vi "氨氮测量流程.vi"(10 "量程模式":T1, 11 "参数":T2={"站号"=1, "量程切换"=enum."AUTO", "控制命令"=enum."启动测量", "模式设置"=enum."待机", "测量间隔"=0} {"站号" items=["总磷"=1, "总氮"=2]}) -> ()   [LabVIEW 2016, in "斯坦道氨氮.lvlib"]
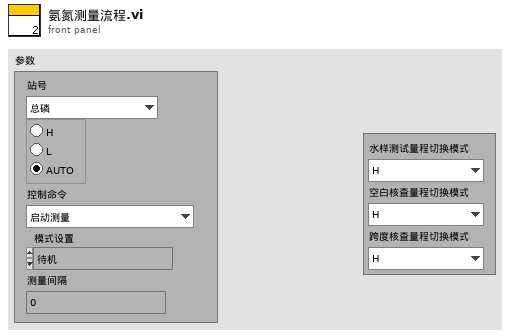
[diagram p1: front panel]
types:
  T1 = cluster{"水样测试量程切换模式":enum16{"H", "L", "AUTO"}, "空白核查量程切换模式":enum16{"H", "L", "AUTO"}, "跨度核查量程切换模式":enum16{"H", "L", "AUTO"}}
  T2 = cluster{"站号":u16, "量程切换":enum32{"H", "L", "AUTO"}, "控制命令":enum16{"启动测量", "标样核查", "零点核查", "跨度核查", "空白测试", "平行样测试", "加标回收", "空白校准", "标样校准", "初始化（清洗）", "停止测试", "仪器重启", "校时", "模式设置", "测量间隔设置"}, "模式设置":enum16{"待机", "连续模式", "周期模式", "定点模式", "受控模式", "手动模式"}, "测量间隔":u16}
  T3 = enum16{"初始化", "通电", "参数1启动", "等待参数1测试完成", "参数1测试完成", "参数1存储数据", "参数2启动", "等待参数2测试完成", "参数2测试完成", "参数2存储数据", "断电", "结束"}
  T4 = cluster{"运行模式":enum16{"维护模式", "常规模式", "应急模式", "质控模式"}, "质控频次":enum16{"关闭", "每天", "星期一", "星期二", "星期三", "星期四", "星期五", "星期六", "星期日"}, "空白核查时间":u16, "跨度核查时间":u16, "24H周期设置":bool[]}
  T5 = cluster{"时间标识":timestamp, "设备":string, "日志信息":string, "流程参数":string}
  T6 = cluster{"时间标识":timestamp, "监测值":sgl, "单位":u16, "数据标识":string, "因子编码":u32, "标样参考值":sgl, "F0":sgl, "F1":sgl, "F2":sgl, "F3":sgl, "温度":sgl, "湿度":sgl, "量程标识":string}
  T7 = enum16{"维护数据", "水样测试", "标样核查", "零点核查", "跨度核查", "空白测试", "平行样测试", "加标回收", "空白校准", "标样校准", "初始化（清洗）"}
  T8 = cluster{"系统时间":timestamp, "工作状态":enum16{"空闲", "水样测试", "标样核查", "零点核查", "跨度核查", "空白测试", "平行样测试", "加标回收", "空白校准", "标样校准", "初始化（清洗）"}, "测量模式":enum16{"待机", "连续模式", "周期模式", "定点模式", "受控模式", "手动模式"}, "告警代码":enum16{"无告警", "缺试剂告警", "缺水样告警", "缺蒸馏水告警", "缺标液告警", "仪表漏液告警", "标定异常告警", "超量程告警", "加热异常", "低试剂预警", "超上限告警", "超下限告警", "仪表内部其他异常", "滴定异常告警", "电极异常告警", "量程切换告警", "参数设置告警", "PH电极电位异常", "电导率电极异常", "浊度光度异常", "溶解氧电极异常", "溶解氧光强异常", "温度异常告警", "PH异常告警", "溶解氧异常告警", "电导率异常告警", "浊度异常告警", "叶绿素异常告警", "藻密度异常告警", "蓝绿藻异常告警", "ORP异常告警", "氨氮异常告警", "清洁刷异常告警", "SD卡异常告警", "蓝牙异常告警", "Wifi异常告警", "流程异常告警"}, "故障代码":enum16{"无故障", "电机故障", "温度故障", "通讯故障", "滴定故障"}, "日志代码":u16, "软件版本":u16, "F0":sgl, "F1":sgl, "F2":sgl, "F3":sgl, "T":sgl, "H":sgl, "id":u16, "flowid":u16, "量程":u16, "总磷控温温度1":sgl, "营养盐控温温度2":sgl, "ADC":sgl}
  T9 = enum16{"启动测量", "标样核查", "零点核查", "跨度核查", "空白测试", "平行样测试", "加标回收", "空白校准", "标样校准", "初始化（清洗）", "停止测试", "仪器重启", "校时", "模式设置", "测量间隔设置"}
  T10 = enum16{"空闲", "水样测试", "标样核查", "零点核查", "跨度核查", "空白测试", "平行样测试", "加标回收", "空白校准", "标样校准", "初始化（清洗）"}
  T11 = cluster{"跨度值":dbl, "零点标准液浓度":dbl, "跨度标准液浓度":dbl, "标准液标准浓度":dbl}
  T12 = cluster{"因子编码":u32, "单位":u16, "标样参考值":sgl, "水样数据时间":timestamp, "水样实测值":sgl, "水样数据标识":string, "标样数据时间":timestamp, "标样实测值":sgl, "标样数据标识":string, "空白数据时间":timestamp, "空白实测值":sgl, "空白数据标识":string, "零点核查数据时间":timestamp, "零点核查实测值":sgl, "零点核查数据标识":string, "跨度核查数据时间":timestamp, "跨度核查实测值":sgl, "跨度核查数据标识":string, "加标回收数据时间":timestamp, "加标回收实测值":sgl, "加标回收数据标识":string, "平行样数据时间":timestamp, "平行样实测值":sgl, "平行样数据标识":string}
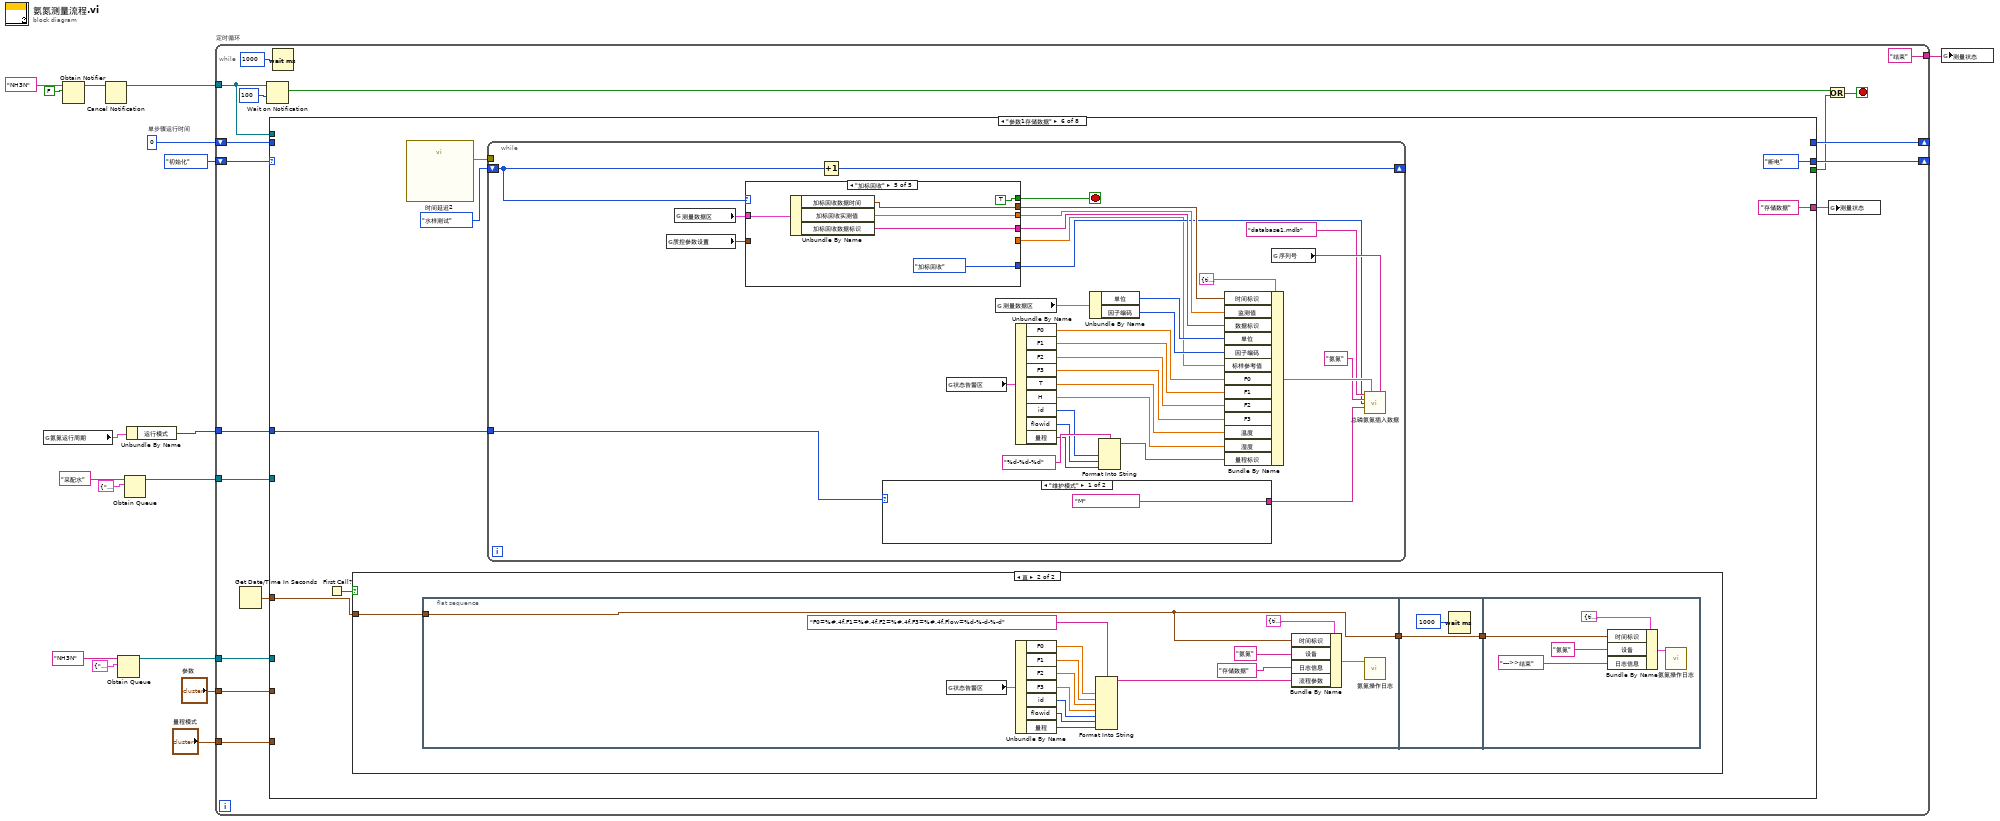
[diagram p0: block diagram]
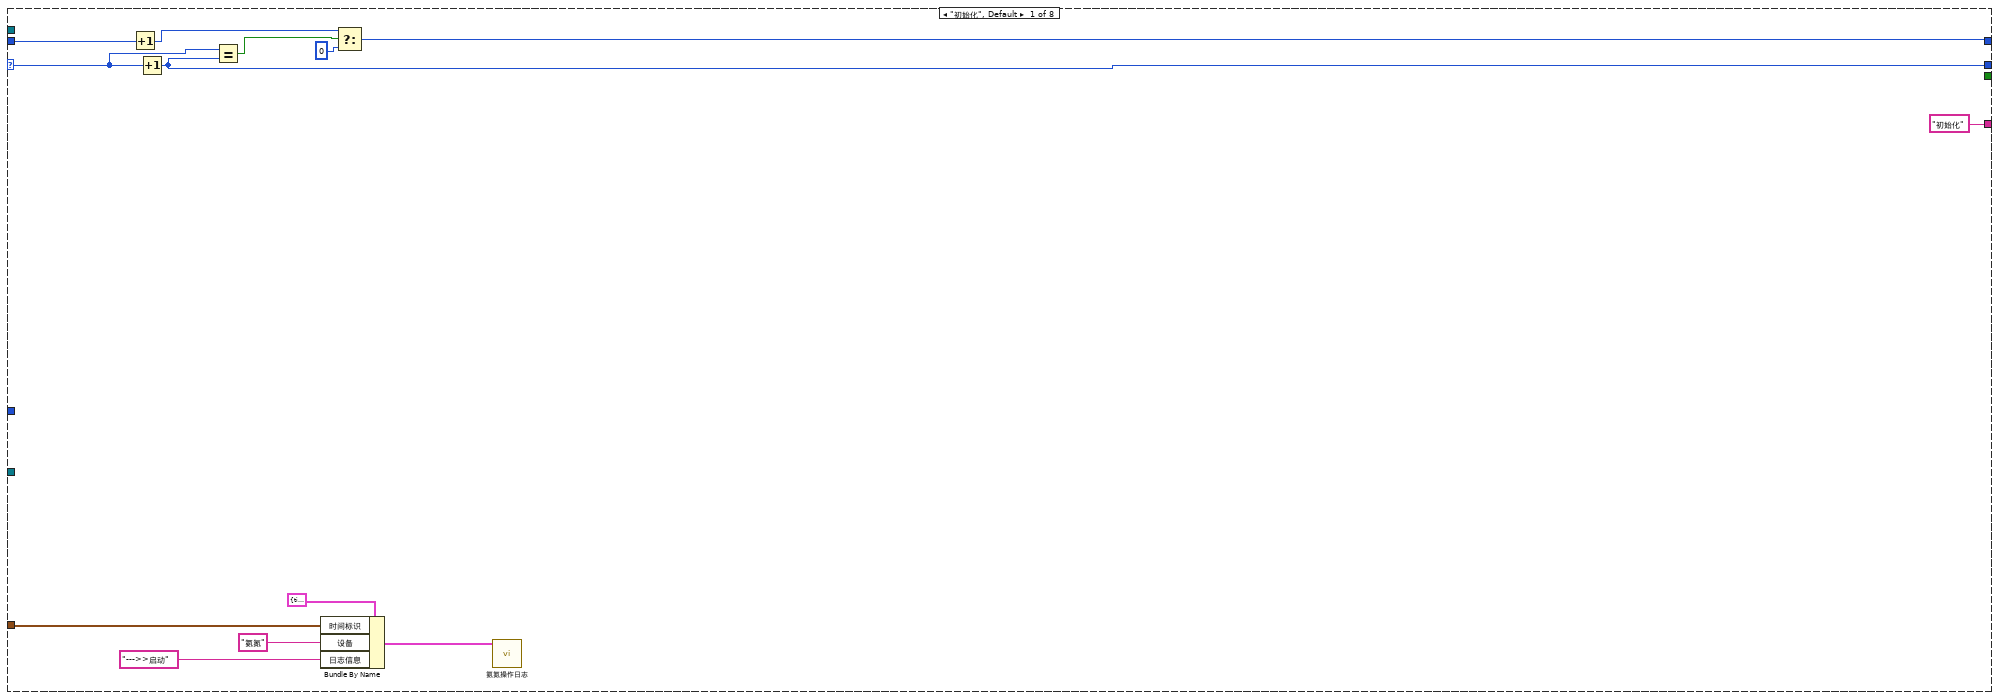
[diagram p2: hidden frame]
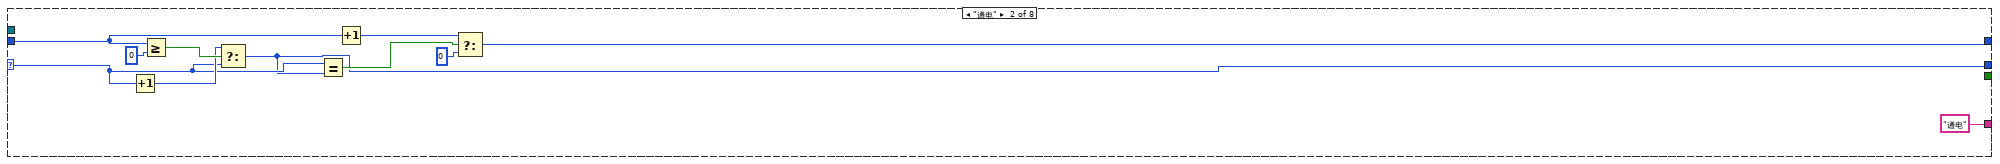
[diagram p3: hidden frame]
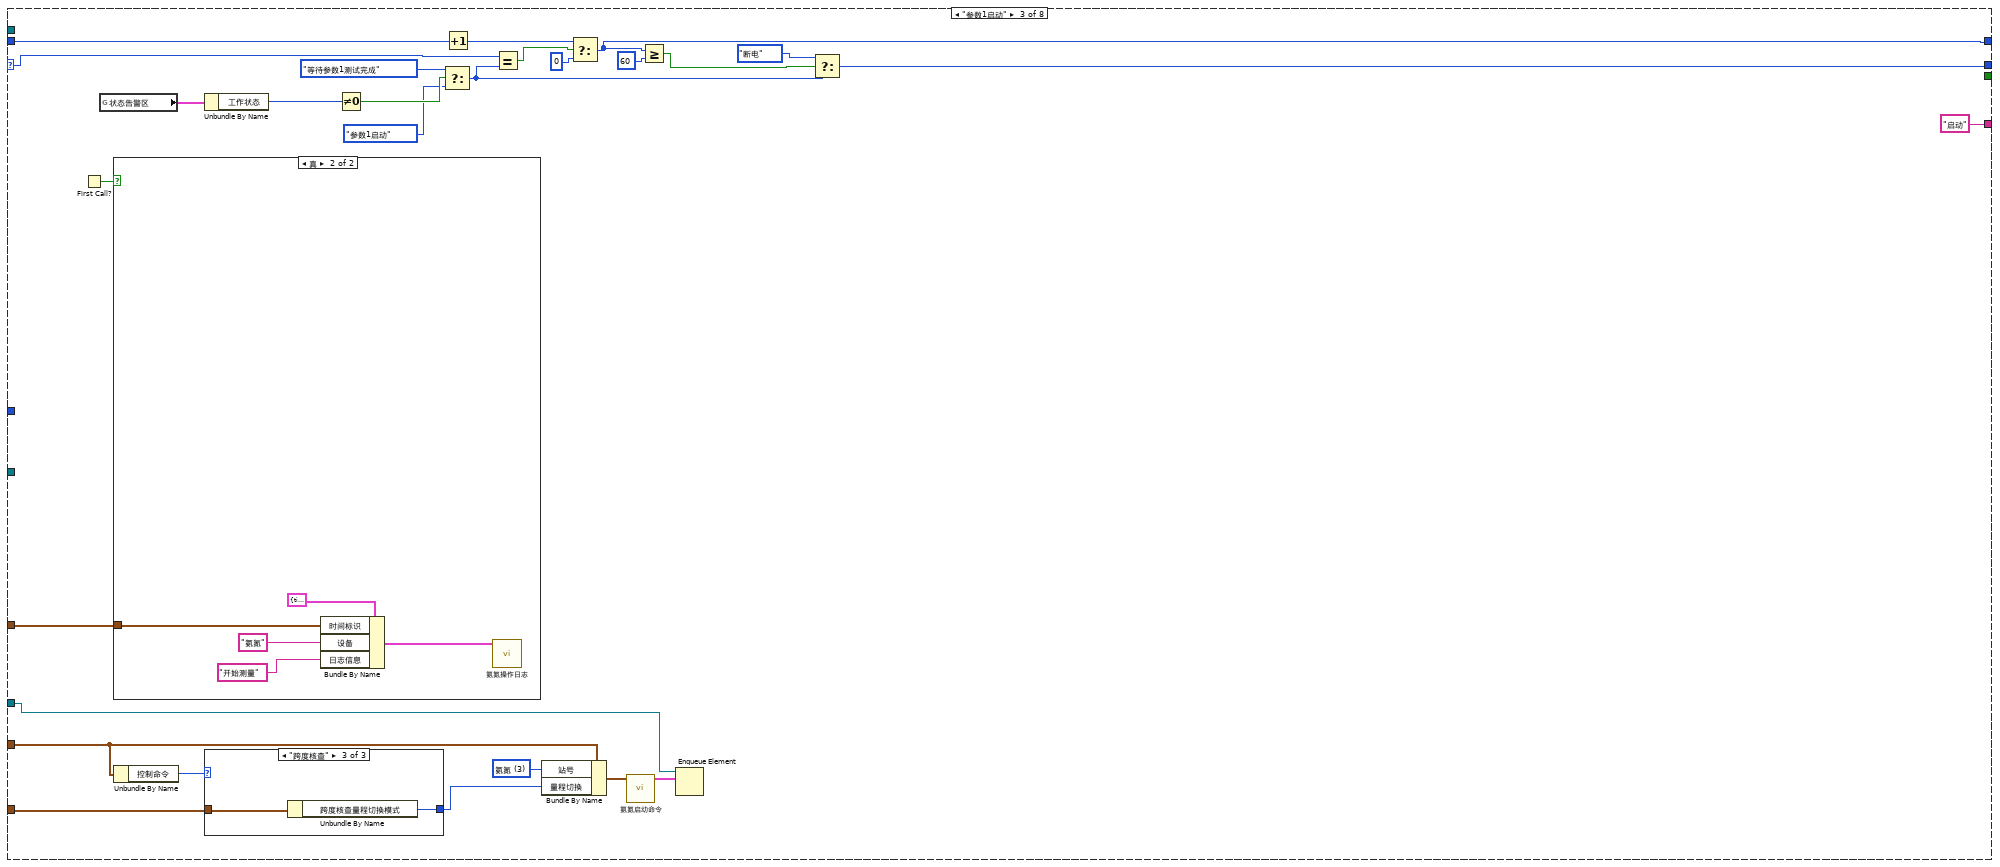
[diagram p4: hidden frame]
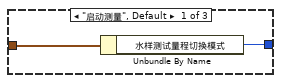
[diagram p5: hidden frame]
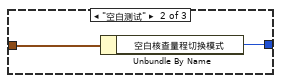
[diagram p6: hidden frame]
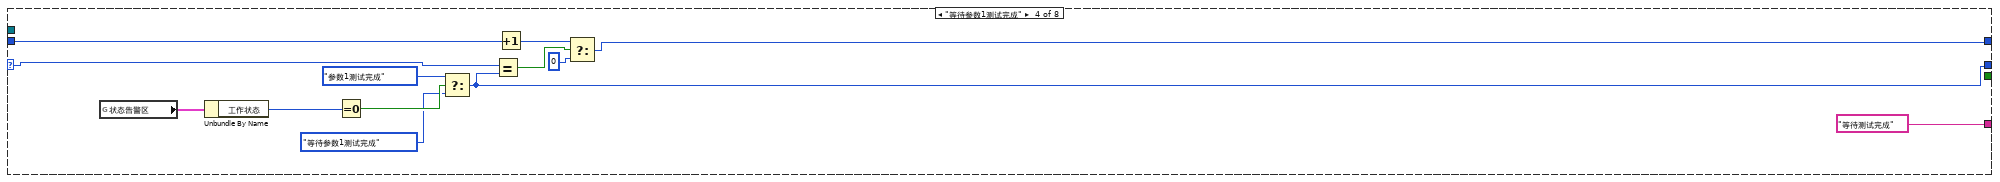
[diagram p8: hidden frame]
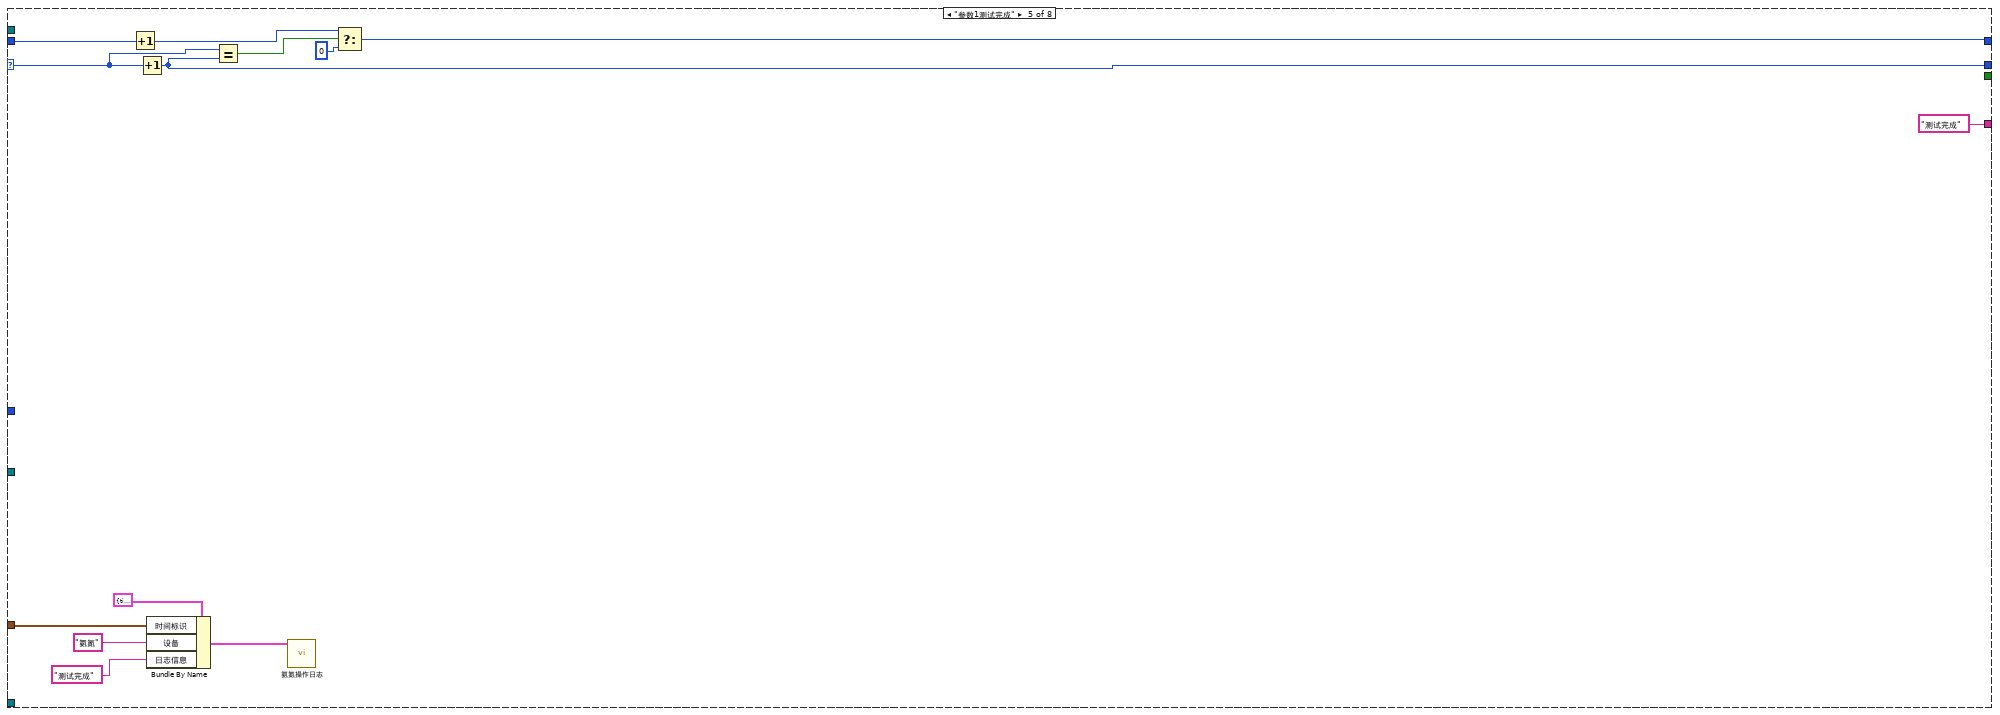
[diagram p9: hidden frame]
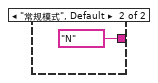
[diagram p10: hidden frame]
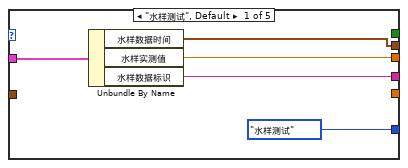
[diagram p11: hidden frame]
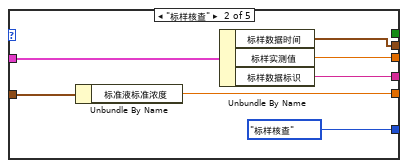
[diagram p12: hidden frame]
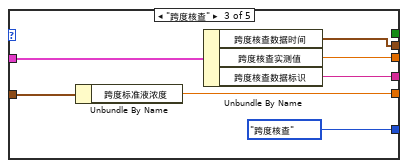
[diagram p13: hidden frame]
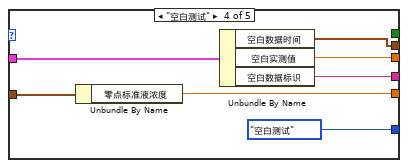
[diagram p14: hidden frame]
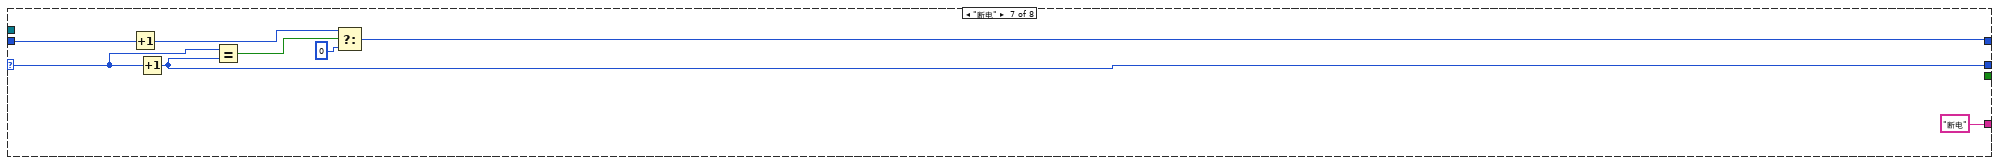
[diagram p16: hidden frame]
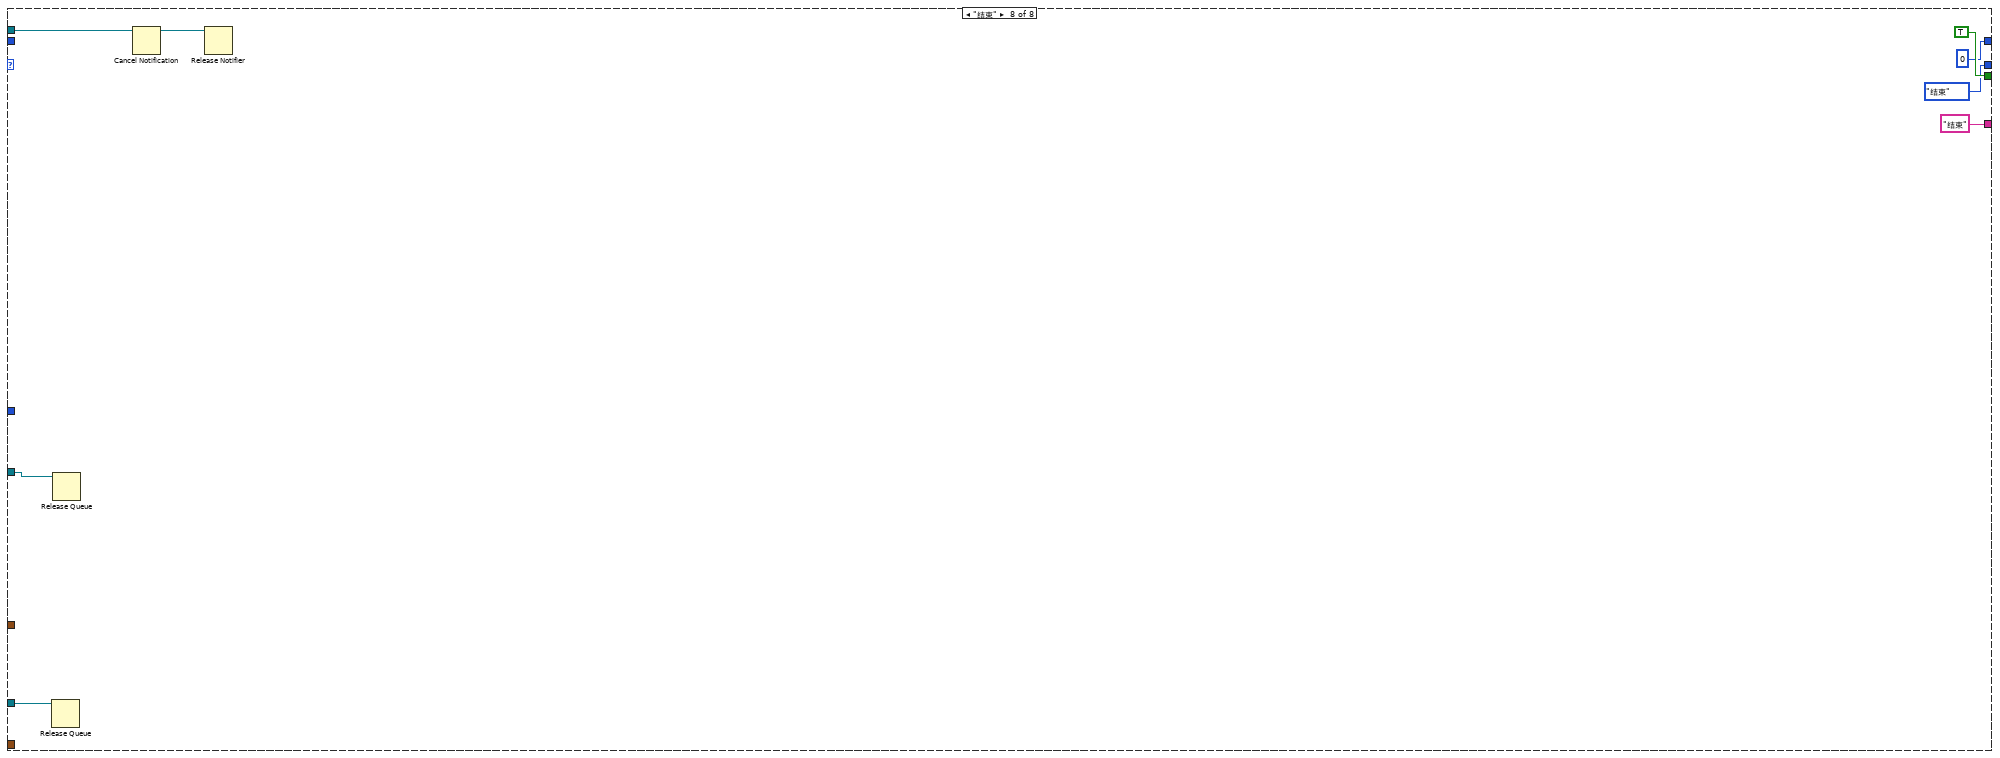
[diagram p17: hidden frame]
diagram:
  w13 = 0  # 单步骤运行时间
  n1 = global read "氨氮断电保存全局变量.vi" "氨氮运行周期"() -> (w2:T4)
  n2 = Obtain Notifier(name (unnamed)="NH3N" ("名称（未命名）"), notification data type=FALSE) -> (notifier out=w10:refnum<notifier>)  [unwired: 2 in, 2 out]
  n3 = Cancel Notification(0:w10) -> (8:w9:refnum<notifier>)  [unwired: 1 in, 2 out]
  n4 = Obtain Queue(name (unnamed)="NH3N" ("名称（未命名）"), element data type=cluster{"命令":string, "data":variant} {"命令"="", "data"=variant}) -> (queue out=w14:refnum<queue>)  [unwired: 3 in, 2 out]
  n5 = Obtain Queue(name (unnamed)="采配水" ("名称（未命名）"), element data type=cluster{"命令":string, "数据":variant} {"命令"="", "数据"=variant}) -> (queue out=w3:refnum<queue>)  [unwired: 3 in, 2 out]
  n6 = Unbundle By Name(w2) -> ("运行模式"=w1:enum16{"维护模式", "常规模式", "应急模式", "质控模式"})
  n7 = while "定时循环" {
    shift-right: [w34] -> _
    shift-left: T3."初始化" ("枚举") -> [w35]
    tunnel: w14 -> [w33]
    shift-right: [w31] -> _
    shift-left: w13 -> [w32]
    tunnel: w9 -> [w30]
    tunnel: "参数" -> [w25]
    tunnel: "量程模式" -> [w22]
    tunnel: ["结束" ("输入 1")] -> w6
    tunnel: w3 -> [w19]
    tunnel: w1 -> [w18]
    stop <- w26 stop-if-true
    n8 = Get Date/Time In Seconds() -> (seconds since 1Jan1904=w23:timestamp)
    n9 = Wait on Notification(notifier=w30, timeout in ms (-1)=100 ("超时毫秒(-1)")) -> (notification=w27:bool)  [unwired: 2 in, 3 out]
    n10 = case shown="\"参数1存储数据\"" w35 {
      selector: w35 -> [w46 w53 w81 w105 w120 _ w227 _]
      tunnel: [_ _ _ _ _ _ _ TRUE] -> w28
      tunnel: [w47 w52 w63 w104 w119 T3."断电" ("枚举") w226 T3."结束" ("枚举")] -> w34
      tunnel: w33 -> [_ _ w86 _ _ _ _ w235]
      tunnel: w32 -> [w48 w54 w82 w107 w121 _ w229 _]
      tunnel: [w44 w55 w68 w106 w122 _ w228 0 ("t")] -> w31
      tunnel: w30 -> [_ _ _ _ _ _ _ w234]
      tunnel: w25 -> [_ _ w72 _ _ _ _ _]
      tunnel: w23 -> [w38 _ w77 _ w113 w130 _ _]
      tunnel: ["初始化" ("输入 1") "通电" ("输入 1") "启动" ("输入 1") "等待测试完成" ("输入 1") "测试完成" ("输入 1") "存储数据" ("输入 1") "断电" ("输入 1") "结束" ("输入 1")] -> w21
      tunnel: w22 -> [_ _ w70 _ _ _ _ _]
      tunnel: w19 -> [_ _ _ _ _ _ _ w230]
      tunnel: w18 -> [_ _ _ _ _ w124 _ _]
      frame "初始化", Default {
        n11 = Increment(x=w48) -> (x+1=w42:i32)
        n12 = Increment(x=w46) -> (x+1=w47:T3)
        n13 = Equal?(x=w46, y=w47) -> (x = y?=w45:bool)
        n14 = Bundle By Name(cluster=T5 {"时间标识"=timestamp(0 s since 1904-01-01), "设备"="", "日志信息"="", "流程参数"=""} ("data in"), "时间标识"=w38, "设备"="氨氮", "日志信息"="--->>启动") -> (w36:T5)
        n15 = Select(t=w42, s=w45, f=0 ("t")) -> (s? t:f=w44:i32)
        n16 = call "氨氮操作日志.vi"("data in"=w36) -> ()  [unwired: 11 in]
      }
      frame "通电" {
        n17 = Increment(x=w53) -> (x+1=w57:T3)
        n18 = Greater Or Equal?(x=w54, y=0) -> (x >= y?=w58:bool)
        n19 = Select(t=w57, s=w58, f=w53) -> (s? t:f=w52:T3)
        n20 = Equal?(x=w53, y=w52) -> (x = y?=w56:bool)
        n21 = Increment(x=w54) -> (x+1=w51:i32)
        n22 = Select(t=w51, s=w56, f=0 ("t")) -> (s? t:f=w55:i32)
      }
      frame "参数1启动" {
        w78 = u16 3 items=["总磷"=1, "总氮"=2, "氨氮"=3] ("站号")
        n23 = First Call?() -> (First Call?: T/F=w76:bool)
        n24 = global read "VAR氨氮全局变量.vi" "状态告警区"() -> (w60:T8)
        n25 = case shown="真" w76 {
          tunnel: w77 -> [_ w94]
          frame False {
          }
          frame True {
            n26 = Bundle By Name(cluster=T5 {"时间标识"=timestamp(0 s since 1904-01-01), "设备"="", "日志信息"="", "流程参数"=""} ("data in"), "时间标识"=w94, "设备"="氨氮", "日志信息"="开始测量") -> (w93:T5)
            n27 = call "氨氮操作日志.vi"("data in"=w93) -> ()  [unwired: 11 in]
          }
        }
        n28 = Unbundle By Name(w72) -> ("控制命令"=w71:T9)
        n29 = Unbundle By Name(w60) -> ("工作状态"=w85:T10)
        n30 = case shown="\"跨度核查\"" w71 {
          tunnel: w70 -> [w88 w90 w92]
          tunnel: [w87 w89 w91] -> w69
          frame "启动测量", Default {
            n31 = Unbundle By Name(w88) -> ("水样测试量程切换模式"=w87:enum16{"H", "L", "AUTO"})
          }
          frame "空白测试" {
            n32 = Unbundle By Name(w90) -> ("空白核查量程切换模式"=w89:enum16{"H", "L", "AUTO"})
          }
          frame "跨度核查" {
            n33 = Unbundle By Name(w92) -> ("跨度核查量程切换模式"=w91:enum16{"H", "L", "AUTO"})
          }
        }
        n34 = Not Equal To 0?(x=w85) -> (x != 0?=w84:bool)
        n35 = Select(t=T3."等待参数1测试完成" ("枚举"), s=w84, f=T3."参数1启动" ("枚举")) -> (s? t:f=w65:T3)
        n36 = Increment(x=w82) -> (x+1=w79:i32)
        n37 = Equal?(x=w81, y=w65) -> (x = y?=w83:bool)
        n38 = Bundle By Name(cluster=w72, "站号"=w78, "量程切换"=w69) -> (w62:T2)
        n39 = Select(t=w79, s=w83, f=0 ("t")) -> (s? t:f=w68:i32)
        n40 = call "氨氮启动命令.vi"("参数"=w62) -> ("启动命令"=w61:cluster{"命令":string, "data":variant})  [unwired: 10 in]
        n41 = Greater Or Equal?(x=w68, y=60) -> (x >= y?=w66:bool)
        n42 = Enqueue Element(queue=w86, element=w61) -> ()  [unwired: 2 in, 3 out]
        n43 = Select(t=T3."断电" ("枚举"), s=w66, f=w65) -> (s? t:f=w63:T3)
      }
      frame "等待参数1测试完成" {
        n44 = global read "VAR氨氮全局变量.vi" "状态告警区"() -> (w98:T8)
        n45 = Unbundle By Name(w98) -> ("工作状态"=w110:T10)
        n46 = Equal To 0?(x=w110) -> (x = 0?=w109:bool)
        n47 = Select(t=T3."参数1测试完成" ("枚举"), s=w109, f=T3."等待参数1测试完成" ("枚举")) -> (s? t:f=w104:T3)
        n48 = Equal?(x=w105, y=w104) -> (x = y?=w108:bool)
        n49 = Increment(x=w107) -> (x+1=w102:i32)
        n50 = Select(t=w102, s=w108, f=0 ("t")) -> (s? t:f=w106:i32)
      }
      frame "参数1测试完成" {
        n51 = Increment(x=w121) -> (x+1=w117:i32)
        n52 = Increment(x=w120) -> (x+1=w119:T3)
        n53 = Bundle By Name(cluster=T5 {"时间标识"=timestamp(0 s since 1904-01-01), "设备"="", "日志信息"="", "流程参数"=""} ("data in"), "时间标识"=w113, "设备"="氨氮", "日志信息"="测试完成") -> (w111:T5)
        n54 = Equal?(x=w120, y=w119) -> (x = y?=w123:bool)
        n55 = call "氨氮操作日志.vi"("data in"=w111) -> ()  [unwired: 11 in]
        n56 = Select(t=w117, s=w123, f=0 ("t")) -> (s? t:f=w122:i32)
      }
      frame "参数1存储数据" {
        n57 = First Call?() -> (First Call?: T/F=w128:bool)
        n58 = case shown="真" w128 {
          tunnel: w130 -> [_ w199]
          frame False {
          }
          frame True {
            n59 = flat-sequence {
              tunnel: w199 -> [w211]
              tunnel: [w211] -> w198
              tunnel: w198 -> [w216]
              tunnel: [w216] -> w197
              tunnel: w197 -> [w218]
              frame #0 {
                n60 = global read "VAR氨氮全局变量.vi" "状态告警区"() -> (w201:T8)
                n61 = Unbundle By Name(w201) -> ("F0"=w203:sgl, "F1"=w204:sgl, "F2"=w205:sgl, "F3"=w206:sgl, "id"=w207:u16, "flowid"=w208:u16, "量程"=w209:u16)
                n62 = Format Into String(format string="F0=%#.4f,F1=%#.4f,F2=%#.4f,F3=%#.4f,Flow=%d-%-d-%-d" ("格式字符串"), w203, w204, w205, w206, w207, w208, w209) -> (resulting string=w202:string)  [unwired: 2 in, 1 out]
                n63 = Bundle By Name(cluster=T5 {"时间标识"=timestamp(0 s since 1904-01-01), "设备"="", "日志信息"="", "流程参数"=""} ("data in"), "时间标识"=w211, "设备"="氨氮", "日志信息"="存储数据", "流程参数"=w202) -> (w200:T5)
                n64 = call "氨氮操作日志.vi"("data in"=w200) -> ()  [unwired: 11 in]
              }
              frame #1 {
                n65 = Wait (ms)(milliseconds to wait=u32 1000 ("等待时间（毫秒）")) -> ()  [unwired: 1 out]
              }
              frame #2 {
                n66 = Bundle By Name(cluster=T5 {"时间标识"=timestamp(0 s since 1904-01-01), "设备"="", "日志信息"="", "流程参数"=""} ("data in"), "时间标识"=w218, "设备"="氨氮", "日志信息"="--->>结束") -> (w217:T5)
                n67 = call "氨氮操作日志.vi"("data in"=w217) -> ()  [unwired: 11 in]
              }
            }
          }
        }
        n68 = call "时间延迟2"() -> ("error out"=w125:errorcluster)  [unwired: 11 in]
        n69 = while {
          shift-right: [w156] -> _
          shift-left: enum16{"水样测试", "标样核查", "跨度核查", "空白测试", "加标回收"}."水样测试" ("测量模式") -> [w157]
          tunnel: w125 -> [_]
          tunnel: w124 -> [w131]
          stop <- w158 stop-if-true
          n70 = global read "氨氮断电保存全局变量.vi" "质控参数设置"() -> (w133:T11)
          n71 = global read "VAR氨氮全局变量.vi" "测量数据区"() -> (w150:T12)
          n72 = case shown="\"加标回收\"" w157 {
            tunnel: w150 -> [w165 w172 w179 w186 w191]
            tunnel: [w169 w176 w183 w190 w196] -> w155
            tunnel: [w168 w175 w182 w189 w195] -> w154
            tunnel: [w167 w174 w181 w188 w194] -> w153
            tunnel: [T7."水样测试" ("测量模式") T7."标样核查" ("测量模式") T7."跨度核查" ("测量模式") T7."空白测试" ("测量模式") T7."加标回收" ("测量模式")] -> w142
            tunnel: [_ _ _ _ TRUE] -> w158
            tunnel: w133 -> [_ w171 w178 w185 _]
            tunnel: [_ w170 w177 w184 _] -> w132
            frame "水样测试", Default {
              n73 = Unbundle By Name(w165) -> ("水样数据时间"=w169:timestamp, "水样实测值"=w168:sgl, "水样数据标识"=w167:string)
            }
            frame "标样核查" {
              n74 = Unbundle By Name(w171) -> ("标准液标准浓度"=w170:dbl)
              n75 = Unbundle By Name(w172) -> ("标样数据时间"=w176:timestamp, "标样实测值"=w175:sgl, "标样数据标识"=w174:string)
            }
            frame "跨度核查" {
              n76 = Unbundle By Name(w178) -> ("跨度标准液浓度"=w177:dbl)
              n77 = Unbundle By Name(w179) -> ("跨度核查数据时间"=w183:timestamp, "跨度核查实测值"=w182:sgl, "跨度核查数据标识"=w181:string)
            }
            frame "空白测试" {
              n78 = Unbundle By Name(w185) -> ("零点标准液浓度"=w184:dbl)
              n79 = Unbundle By Name(w186) -> ("空白数据时间"=w190:timestamp, "空白实测值"=w189:sgl, "空白数据标识"=w188:string)
            }
            frame "加标回收" {
              n80 = Unbundle By Name(w191) -> ("加标回收数据时间"=w196:timestamp, "加标回收实测值"=w195:sgl, "加标回收数据标识"=w194:string)
            }
          }
          n81 = Increment(x=w157) -> (x+1=w156:enum16{"水样测试", "标样核查", "跨度核查", "空白测试", "加标回收"})
          n82 = case shown="\"维护模式\"" w131 {
            tunnel: ["M" ("数据标记表") "N" ("数据标记表")] -> w134
            frame "维护模式" {
            }
            frame "常规模式", Default {
            }
          }
          n83 = global read "VAR氨氮全局变量.vi" "状态告警区"() -> (w148:T8)
          n84 = global read "VAR氨氮全局变量.vi" "测量数据区"() -> (w149:T12)
          n85 = Unbundle By Name(w148) -> ("F0"=w140:sgl, "F1"=w139:sgl, "F2"=w138:sgl, "F3"=w137:sgl, "T"=w136:sgl, "H"=w135:sgl, "id"=w161:u16, "flowid"=w160:u16, "量程"=w159:u16)
          n86 = Unbundle By Name(w149) -> ("单位"=w152:u16, "因子编码"=w151:u32)
          n87 = Format Into String(format string="%d-%d-%d" ("格式字符串"), w161, w160, w159) -> (resulting string=w141:string)  [unwired: 2 in, 1 out]
          n88 = Bundle By Name(cluster=T6 {"时间标识"=timestamp(0 s since 1904-01-01), "监测值"=0.0, "单位"=0, "数据标识"="", "因子编码"=0, "标样参考值"=0.0, "F0"=0.0, "F1"=0.0, "F2"=0.0, "F3"=0.0, "温度"=0.0, "湿度"=0.0, "量程标识"=""} ("data"), "时间标识"=w155, "监测值"=w154, "数据标识"=w153, "单位"=w152, "因子编码"=w151, "标样参考值"=w132, "F0"=w140, "F1"=w139, "F2"=w138, "F3"=w137, "温度"=w136, "湿度"=w135, "量程标识"=w141) -> (w146:T6)
          n89 = global read "VAR氨氮全局变量.vi" "序列号"() -> (w145:string)
          n90 = call "总磷氨氮插入数据.vi"("database"="database1.mdb", "data"=w146, "SN"=w145, "table"="氨氮", "测量模式"=w142, "数据标记表"=w134) -> ()  [unwired: 9 in, 1 out]
        }
      }
      frame "断电" {
        n91 = Increment(x=w229) -> (x+1=w222:i32)
        n92 = Increment(x=w227) -> (x+1=w226:T3)
        n93 = Equal?(x=w227, y=w226) -> (x = y?=w224:bool)
        n94 = Select(t=w222, s=w224, f=0 ("t")) -> (s? t:f=w228:i32)
      }
      frame "结束" {
        n95 = Release Queue(queue=w235) -> ()  [unwired: 2 in, 3 out]
        n96 = Release Queue(queue=w230) -> ()  [unwired: 2 in, 3 out]
        n97 = Cancel Notification(0:w234) -> (8:w233:refnum<notifier>)  [unwired: 1 in, 2 out]
        n98 = Release Notifier(notifier=w233) -> ()  [unwired: 2 in, 3 out]
      }
    }
    n99 = Wait (ms)(milliseconds to wait=u32 1000 ("等待时间（毫秒）")) -> ()  [unwired: 1 out]
    n100 = Or(x=w27, y=w28) -> (x .or. y?=w26:bool)
    n101 = global write "VAR氨氮全局变量.vi" "测量状态"(w21) -> ()
  }
  n102 = global write "VAR氨氮全局变量.vi" "测量状态"(w6) -> ()
